vi "Set_Installer.vi"(8 "error in (no error)":errorcluster, 10 "data":T1={"Destination"=[], "Source"=[], "buildObject"=0, "defaultDir"="", "platform"="", "author"="", "productName"="", "buildSpecName"="", "hide"=FALSE, "requireLVDevSys"=FALSE, "autoIncrement"=FALSE, "includeError"=FALSE, "readmeID"="", "buildLocation"=path "", "readmePath"=path "", "mediaSize"=0, "language"=9, "productVersion"={"Major"=1, "Minor"=0, "Update"=0}, "preview"=FALSE, "programmatic"=FALSE, "progressBarEvents"={"newJob"=refnum, "newItem"=refnum, "errorMsg"=refnum, "cancel"=refnum}, "userLog_Path"=path "", "shortcutAddresses"=[], "EXE_Install Address"="", "EXE_Uninstall Address"="", "additional NIPaths"=[], "web service itemIDs"=[], "installerName"=""} {"productVersion"."Update" step=1; "productVersion"."Minor" step=1; "productVersion"."Major" step=1; "language" items=["English"=9, "German"=7, "French"=12, "Japanese"=17, "Korean"=18, "Chinese (Simplified)"=2052]}, 11 "Installer in":refnum<class "Installer.lvclass">) -> (0 "error out":errorcluster, 3 "Installer out":refnum<class "Installer.lvclass">)   [LabVIEW 2020, in "Installer.lvclass"]
uses:
  <vilib>/AppBuilder/IB_Classes/Installer/Installer.lvclass
  <vilib>/AppBuilder/IB_Classes/Installer/Installer.lvclass/Installer.ctl
  <resource>/Framework/Providers/Builds/Installer/CDK_sTypeDef_Languages.ctl
  <resource>/Framework/Providers/Builds/Installer/CDK_sTypeDef_ProductVersion.ctl
  <resource>/Framework/Providers/API/ItemRef.ctl
  <resource>/Framework/Providers/API/mxLvBuildError.ctl
  <resource>/Framework/Providers/Common/provcom_ProgressBar_Events.ctl
  <vilib>/AppBuilder/IB_Classes/Destination/IB_Destination.lvclass
  <vilib>/AppBuilder/IB_Classes/Installer/IB_Installer.ctl
  <vilib>/AppBuilder/IB_Classes/Source/IB_Source.lvclass
  <resource>/Framework/Providers/Builds/Installer/CDK_sTypeDef_ShortcutAddress.ctl
  <vilib>/AppBuilder/IB_Classes/Dest_NI_NIPath/Dest_NI_NIPath.lvclass
panel:
  # "."
  # "."
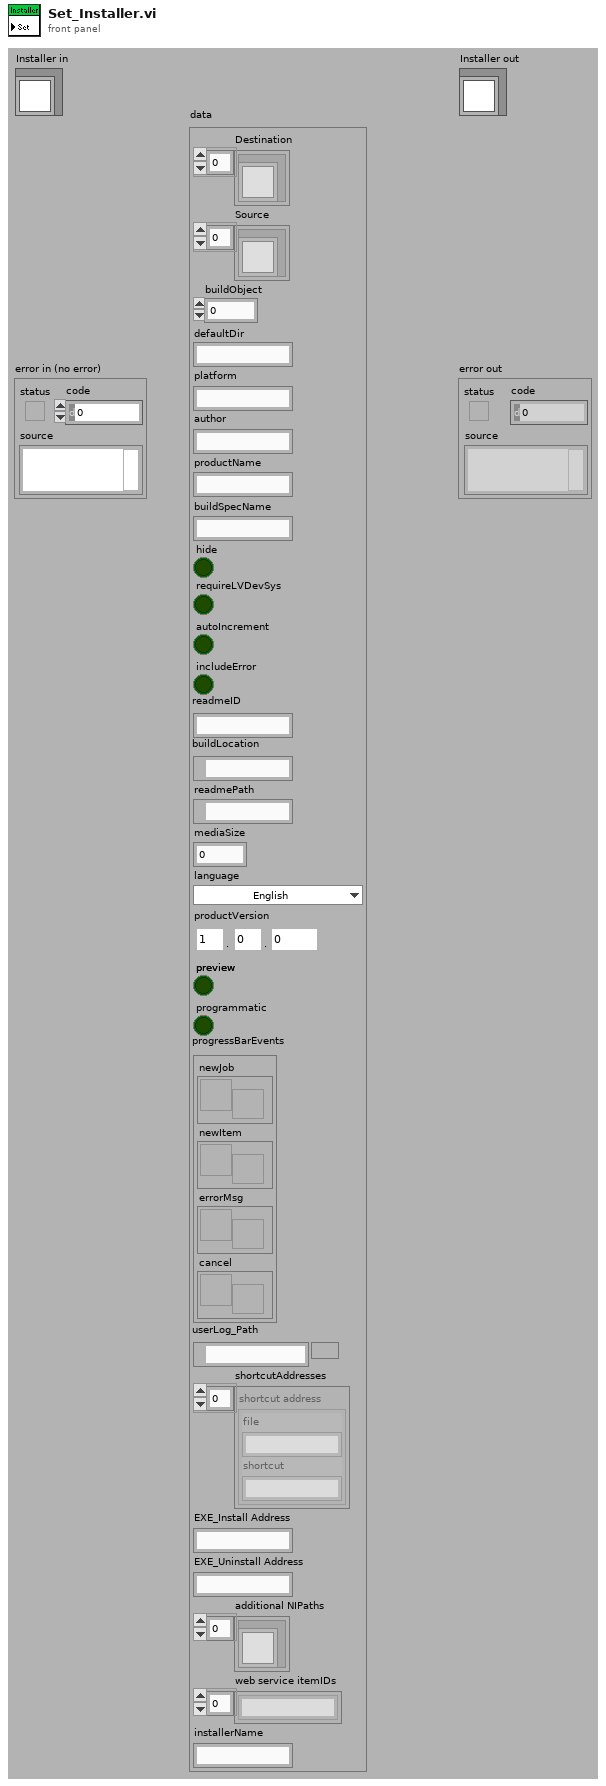
[diagram p1: front panel]
types:
  T1 = typedef "IB_Installer.ctl" = cluster{"Destination":refnum<class "IB_Destination.lvclass">[], "Source":refnum<class "IB_Source.lvclass">[], "buildObject":T2, "defaultDir":string, "platform":string, "author":string, "productName":string, "buildSpecName":string, "hide":bool, "requireLVDevSys":bool, "autoIncrement":bool, "includeError":bool, "readmeID":string, "buildLocation":path, "readmePath":path, "mediaSize":u16, "language":T3, "productVersion":T4, "preview":bool, "programmatic":bool, "progressBarEvents":T5, "userLog_Path":path, "shortcutAddresses":T7[], "EXE_Install Address":string, "EXE_Uninstall Address":string, "additional NIPaths":refnum<class "Dest_NI_NIPath.lvclass">[], "web service itemIDs":string[], "installerName":string}
  T2 = typedef "ItemRef.ctl" = u64
  T3 = typedef "CDK_sTypeDef_Languages.ctl" = u16
  T4 = typedef "CDK_sTypeDef_ProductVersion.ctl" = cluster{"Major":u8, "Minor":u8, "Update":u16}
  T5 = typedef "provcom_ProgressBar_Events.ctl" = cluster{"newJob":refnum<user-event>, "newItem":refnum<user-event>, "errorMsg":T6, "cancel":refnum<user-event>}
  T6 = typedef "mxLvBuildError.ctl" = refnum<user-event>
  T7 = typedef "CDK_sTypeDef_ShortcutAddress.ctl" = cluster{"file":string, "shortcut":string}
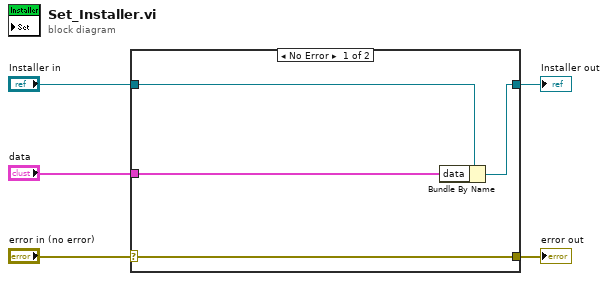
[diagram p0: block diagram]
diagram:
  n1 = case shown="No Error" "error in (no error)" {
    selector: "error in (no error)" -> [w9 w10]
    tunnel: [w9 w10] -> w4
    tunnel: [w7 w11] -> w2
    tunnel: "Installer in" -> [w8 w11]
    tunnel: "data" -> [w6 _]
    frame No Error {
      n2 = Bundle By Name(cluster=w8, "data"=w6) -> (w7:refnum<class "Installer.lvclass">)
    }
    frame Error {
    }
  }
  "error out" <- w4
  "Installer out" <- w2
